vi "GEOM_ParseOverridePars.vi"(6 "override keyword":string, 7 "override comment":string, 8 "keyword in":string, 9 "override pars":string, 10 "section in":string, 11 "comment in":string) -> (0 "keyword out":string, 2 "section out":string, 3 "comment out":string)   [LabVIEW 2016]
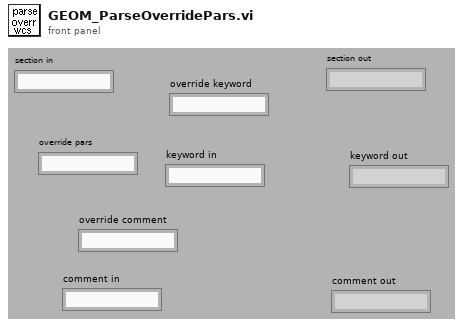
[diagram p1: front panel]
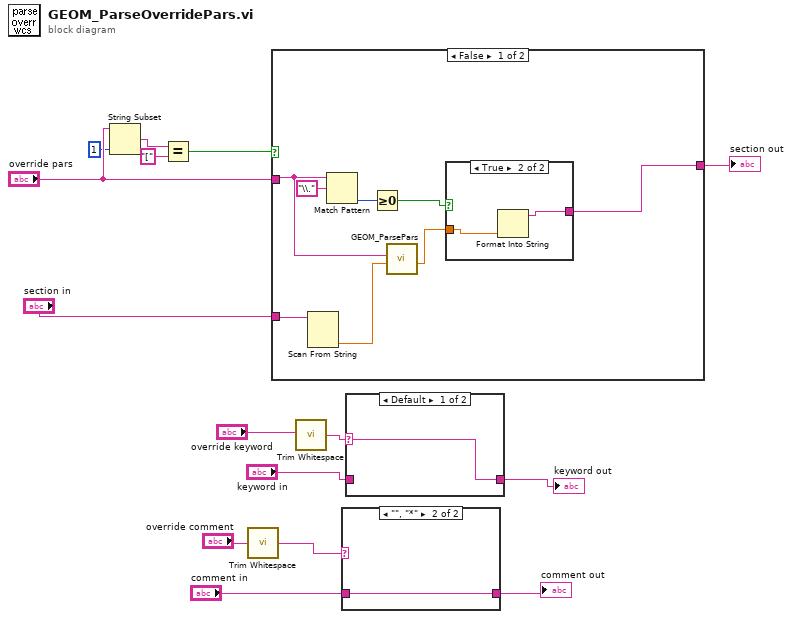
[diagram p0: block diagram]
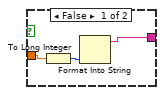
[diagram p3: hidden frame]
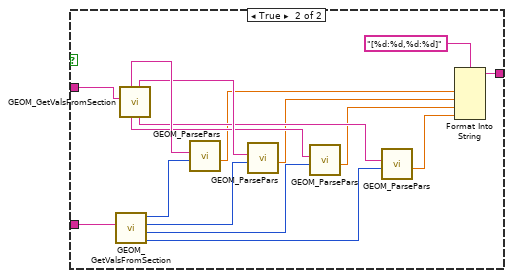
[diagram p4: hidden frame]
diagram:
  n1 = String Subset(string="override pars", length (rest)=1 ("length (rest)")) -> (substring=w7:string)  [unwired: 1 out]
  n2 = Equal?(x=w7, y="[") -> (x = y?=w5:bool)
  n3 = call <vilib>:"Trim Whitespace.vi"("string"="override comment") -> ("trimmed string"=w12:string)  [unwired: 1 in]
  n4 = case shown="False" w5 {
    tunnel: "section in" -> [w23 w44]
    tunnel: [w20 w30] -> w14
    tunnel: "override pars" -> [w18 w29]
    frame False {
      n5 = Scan From String(input string=w23) -> (output 1=w22:dbl)  [unwired: 3 in, 4 out]
      n6 = Match Pattern(string=w18, regular expression="\\.") -> (offset past match=w17:i32)  [unwired: 4 out]
      n7 = Greater Or Equal To 0?(x=w17) -> (x >= 0?=w16:bool)
      n8 = call "GEOM_ParsePars.vi"("ref val"=w22, "par in"=w18) -> ("val out"=w21:dbl)  [unwired: 9 out]
      n9 = case shown="True" w16 {
        tunnel: w21 -> [w26 w27]
        tunnel: [w25 w28] -> w20
        frame False {
          n10 = To Long Integer(number=w26) -> (32bit integer=w24:i32)
          n11 = Format Into String(w24) -> (resulting string=w25:string)  [unwired: 3 in, 1 out]
        }
        frame True {
          n12 = Format Into String(w27) -> (resulting string=w28:string)  [unwired: 3 in, 1 out]
        }
      }
    }
    frame True {
      n13 = call "GEOM_GetValsFromSection.vi"("section"=w44) -> ("yend"=w36:i32, "ystart"=w38:i32, "xend"=w40:i32, "xstart"=w42:i32)  [unwired: 7 out]
      n14 = call "GEOM_GetValsFromSection.vi"("section"=w29) -> ("ye str"=w37:string, "xe str"=w41:string, "ys str"=w39:string, "xs str"=w43:string)  [unwired: 7 out]
      n15 = call "GEOM_ParsePars.vi"("ref val"=w42, "par in"=w43) -> ("val out"=w34:dbl)  [unwired: 9 out]
      n16 = call "GEOM_ParsePars.vi"("ref val"=w40, "par in"=w41) -> ("val out"=w33:dbl)  [unwired: 9 out]
      n17 = call "GEOM_ParsePars.vi"("ref val"=w38, "par in"=w39) -> ("val out"=w32:dbl)  [unwired: 9 out]
      n18 = call "GEOM_ParsePars.vi"("ref val"=w36, "par in"=w37) -> ("val out"=w31:dbl)  [unwired: 9 out]
      n19 = Format Into String(format string="[%d:%d,%d:%d]", w34, w33, w32, w31) -> (resulting string=w30:string)  [unwired: 2 in, 1 out]
    }
  }
  "section out" <- w14
  n20 = call <vilib>:"Trim Whitespace.vi"("string"="override keyword") -> ("trimmed string"=w4:string)  [unwired: 1 in]
  n21 = case shown="\"\", \"*\"" w12 {
    selector: w12 -> [w45 _]
    tunnel: "comment in" -> [_ w46]
    tunnel: [w45 w46] -> w10
    frame Default {
    }
    frame "", "*" {
    }
  }
  "comment out" <- w10
  n22 = case shown="Default" w4 {
    selector: w4 -> [w47 _]
    tunnel: "keyword in" -> [_ w48]
    tunnel: [w47 w48] -> w1
    frame Default {
    }
    frame "", "*" {
    }
  }
  "keyword out" <- w1
